vi "Scan.vi"() -> ()   [LabVIEW 2015]
uses:
  oskar_tools/seq_line.ctl
  oskar_tools/oskar_tools.lvlib
panel:
  in  "Open Button":bool
  in  "Make":bool
  in  "Tab Control":enum32{"Template", "Values", "Output", "README"}(tab)
  in  "Template":T1 caption="Template (placeholder: MOD)"
  in  "build mode":enum32{"step", "array"}(radio)
  in  "Shuffle":bool
  in  "Build Array":bool
  out "Array":string[](array[string])
  in  "Step":dbl=0.1
  in  "Stop":dbl=1.0
  in  "Start":dbl
  in  "Array size":i32=11
  in  "format string":string="%.4g"
  in  "SEQs":T1[](array[typedef])
  in  "Template":T1[](array[typedef])
  out "#":i32
  in  "Save":path
  in  "Stop Button":bool
  in  "Save Button":bool
  in  "Send Button":bool
  in  "New Button":bool
  # "Scan"
  # "### Overview ###\n\nCreate a sequence file that scans a VAR value over a linear series.\n\n### Instructions ###\n\nLoad or create a template sequence, using \"MOD\" in place of the value of the VAR to scan.\n\nOn the \"Values\" tab, build an array to cover the values that the VAR should take during the measurement.\n\nPress \"Make\" to create the sequence.  \"Save\" as a *.jsq file and \"Send\" it to sequencer.vi."
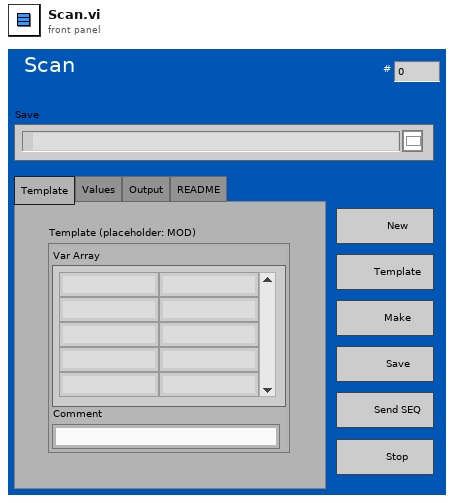
[diagram p1: front panel]
types:
  T1 = typedef "oskar_tools.lvlib/seq_line.ctl" = cluster{"Var Array":string[][], "Comment":string}
  T2 = enum8{"Enabled", "Disabled", "Disabled and Grayed Out"}
  T3 = enum16{"Left Button", "Center Button", "Right Button", "Window Close"}
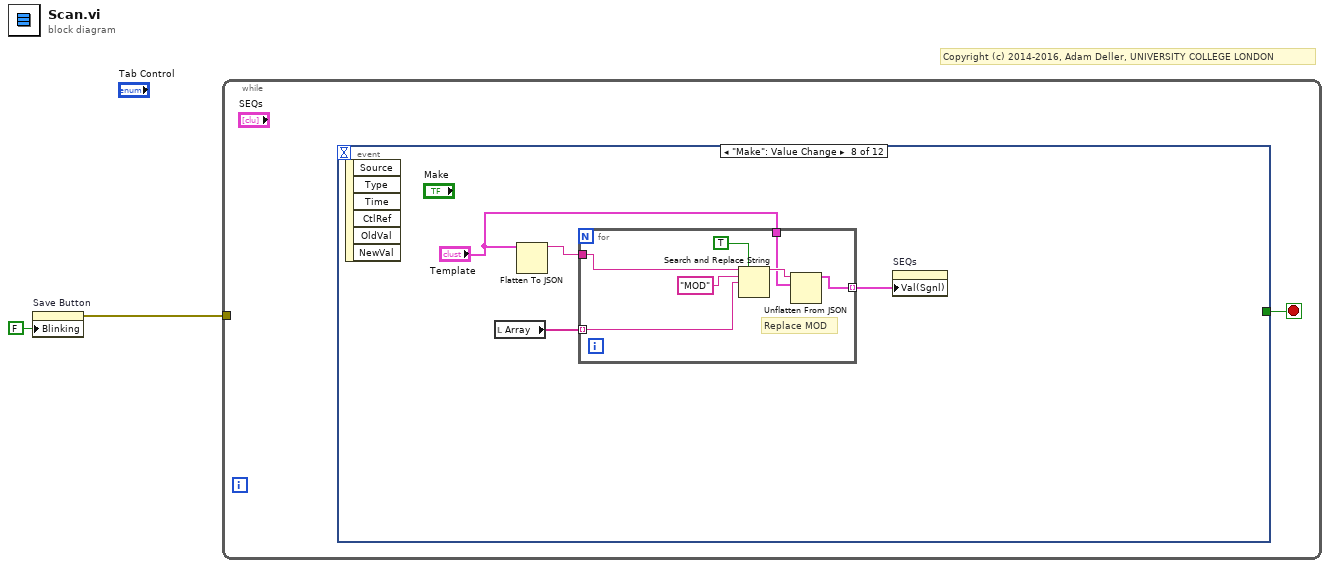
[diagram p0: block diagram]
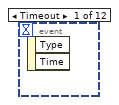
[diagram p2: hidden frame]
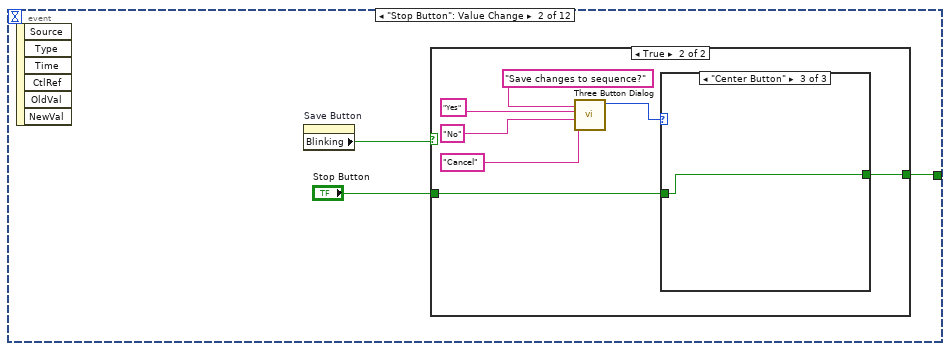
[diagram p3: hidden frame]
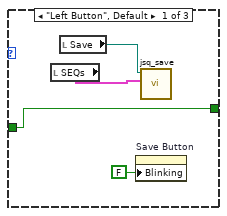
[diagram p5: hidden frame]
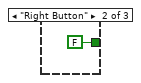
[diagram p6: hidden frame]
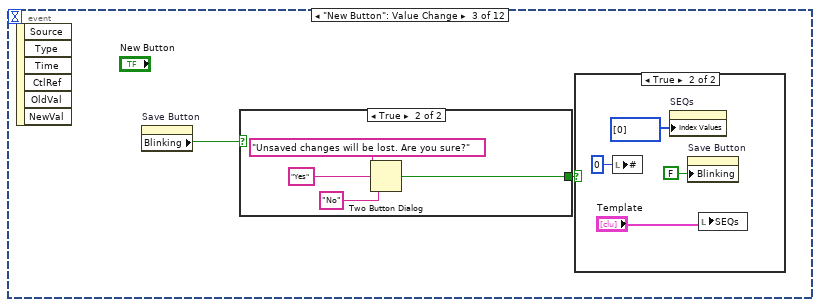
[diagram p7: hidden frame]
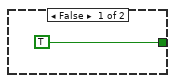
[diagram p9: hidden frame]
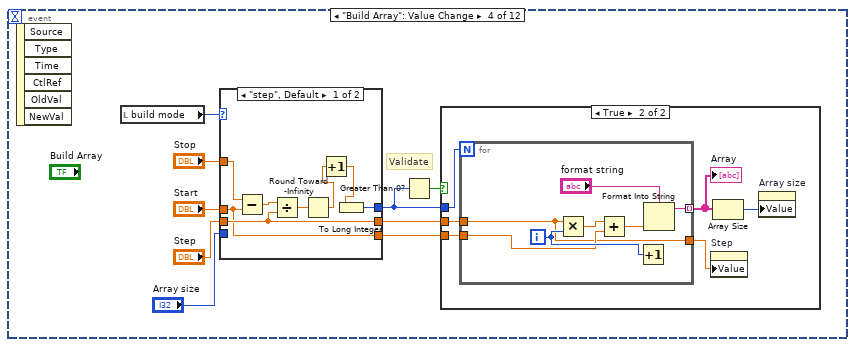
[diagram p10: hidden frame]
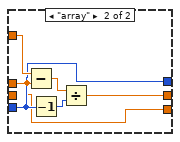
[diagram p11: hidden frame]
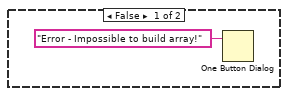
[diagram p12: hidden frame]
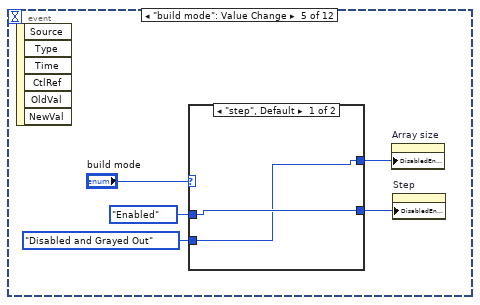
[diagram p13: hidden frame]
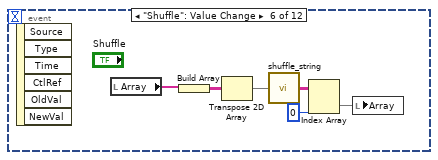
[diagram p15: hidden frame]
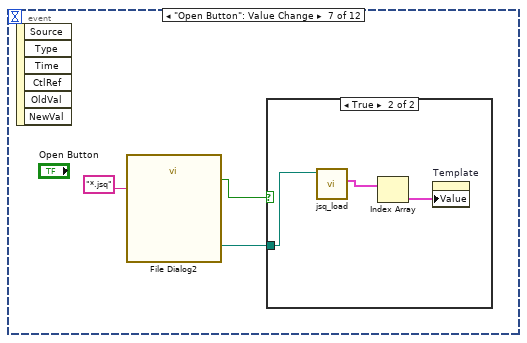
[diagram p16: hidden frame]
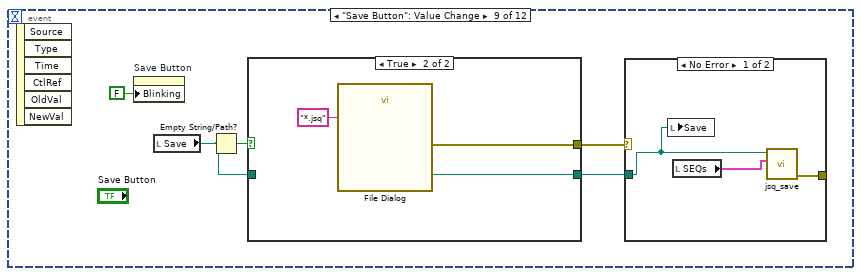
[diagram p18: hidden frame]
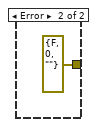
[diagram p19: hidden frame]
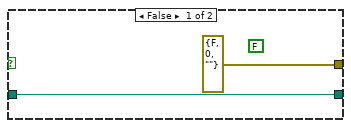
[diagram p20: hidden frame]
diagram:
  # "Copyright (c) 2014-2016, Adam Deller, UNIVERSITY COLLEGE LONDON"
  n1 = property on="Save Button" class="Bool"("Blinking"=FALSE) -> (error out=w1:errorcluster)  [unwired: 2 in, 1 out]
  n2 = while {
    tunnel: w1 -> [_]
    stop <- w3 stop-if-true
    n3 = event shown="[7] \"Make\": Value Change" {
      selector: _ -> [_ _ _ _ _ _ _ _ _ _ _ _]
      dyn-events: _ -> [_ _ _ _ _ _ _ _ _ _ _ _]
      timeout: _ -> [_ _ _ _ _ _ _ _ _ _ _ _]
      tunnel: [_ w6 _ _ _ _ _ _ _ _ _ _] -> w3
      event Timeout {
        n4 = event-data() -> ()  [unwired: 1 in, 2 out]
      }
      event "Stop Button": Value Change {
        n5 = event-data() -> ()  [unwired: 1 in, 6 out]
        n6 = property on="Save Button" class="Bool"() -> ("Blinking"=w5:bool)  [unwired: 2 in, 2 out]
        n7 = case shown="True" w5 {
          tunnel: [w7 w8] -> w6
          tunnel: "Stop Button" -> [w7 w9]
          frame False {
          }
          frame True {
            n8 = call <vilib>:"Three Button Dialog.vi"("Right Button Text (\"Cancel\")"="Cancel" ("Right Button Text (\"Cancel\")"), "Center Button Text (\"No\")"="No" ("F button name (\"Cancel\")"), "Left Button Text (\"Yes\")"="Yes" ("T button name (\"OK\")"), "message"="Save changes to sequence?") -> ("Which Button?"=w10:T3)  [unwired: 7 in]
            n9 = case shown="\"Center Button\"" w10 {
              tunnel: w9 -> [w18 _ w20]
              tunnel: [w18 FALSE ("Stop Button") w20] -> w8
              frame "Left Button", Default {
                n10 = local read "SEQs"() -> (w15:T1[])
                n11 = local read "Save"() -> (w17:path)
                n12 = property on="Save Button" class="Bool"("Blinking"=FALSE) -> ()  [unwired: 2 in, 2 out]
                n13 = call "jsq_save.vi"("SEQs"=w15, "Path"=w17) -> ()  [unwired: 7 in, 3 out]
              }
              frame "Right Button" {
              }
              frame "Center Button" {
              }
            }
          }
        }
      }
      event "New Button": Value Change {
        n14 = event-data() -> ()  [unwired: 1 in, 6 out]
        n15 = property on="Save Button" class="Bool"() -> ("Blinking"=w21:bool)  [unwired: 2 in, 2 out]
        n16 = case shown="True" w21 {
          tunnel: [TRUE w28] -> w22
          frame False {
          }
          frame True {
            n17 = Two Button Dialog(message="Unsaved changes will be lost. Are you sure?", 1:"No" ("F button name (\"Cancel\")"), 2:"Yes" ("T button name (\"OK\")")) -> (T button?=w28:bool)
          }
        }
        n18 = case shown="True" w22 {
          frame False {
          }
          frame True {
            n19 = local write "#"(0 ("#")) -> ()
            n20 = property on="SEQs" class="Arr (strict)"("Index Values"=u32[] [0]) -> ()  [unwired: 2 in, 2 out]
            n21 = property on="Save Button" class="Bool"("Blinking"=FALSE) -> ()  [unwired: 2 in, 2 out]
            n22 = local write "SEQs"("Template") -> ()
          }
        }
      }
      event "Build Array": Value Change {
        # "Validate"
        n23 = event-data() -> ()  [unwired: 1 in, 6 out]
        n24 = local read "build mode"() -> (w33:enum32{"step", "array"})
        n25 = case shown="\"step\", Default" w33 {
          tunnel: "Step" -> [w45 _]
          tunnel: "Stop" -> [w44 w53]
          tunnel: [w43 w49] -> w38
          tunnel: "Start" -> [w43 w49]
          tunnel: "Array size" -> [_ w50]
          tunnel: [w45 w52] -> w37
          tunnel: [w47 w50] -> w39
          frame "step", Default {
            n26 = Subtract(x=w44, y=w43) -> (x-y=w48:dbl)
            n27 = Divide(x=w48, y=w45) -> (x/y=w46:dbl)
            n28 = Round Toward -Infinity(1:w46) -> (0:w42:dbl)
            n29 = Increment(x=w42) -> (x+1=w41:dbl)
            n30 = To Long Integer(number=w41) -> (32bit integer=w47:i32)
          }
          frame "array" {
            n31 = Subtract(x=w53, y=w49) -> (x-y=w54:dbl)
            n32 = Decrement(x=w50) -> (x-1=w51:i32)
            n33 = Divide(x=w54, y=w51) -> (x/y=w52:dbl)
          }
        }
        n34 = Greater Than 0?(x=w39) -> (x > 0?=w40:bool)
        n35 = case shown="True" w40 {
          tunnel: w38 -> [_ w61]
          tunnel: w37 -> [_ w58]
          tunnel: w39 -> [_ w57]
          frame False {
            n36 = One Button Dialog(message="Error - Impossible to build array!") -> ()  [unwired: 1 in, 1 out]
          }
          frame True {
            n37 = for {
              N: w57 -> [_]
              tunnel: w61 -> [w64]
              tunnel: [w65] -> w60 mode=indexing
              tunnel: w58 -> [w62]
              tunnel: [w62] -> w56
              i -> [w68]
              n38 = Multiply(x=w62, y=w68) -> (x*y=w63:dbl)
              n39 = Add(x=w63, y=w64) -> (x+y=w66:dbl)
              n40 = Increment(x=w68) -> ()  [unwired: 1 out]
              n41 = Format Into String(format string="format string", w66) -> (resulting string=w65:string)  [unwired: 2 in, 1 out]
            }
            "Array" <- w60
            n42 = property on="Step" class="DigNum (strict)"("Value"=w56) -> ()  [unwired: 2 in, 2 out]
            n43 = Array Size(array=w60) -> (size(s)=w59:i32)
            n44 = property on="Array size" class="DigNum (strict)"("Value"=w59) -> ()  [unwired: 2 in, 2 out]
          }
        }
      }
      event "build mode": Value Change {
        n45 = event-data() -> ()  [unwired: 1 in, 6 out]
        n46 = case shown="\"step\", Default" "build mode" {
          tunnel: [w74 w77] -> w72
          tunnel: T2."Enabled" ("Disabled") -> [w75 w77]
          tunnel: [w75 w76] -> w70
          tunnel: T2."Disabled and Grayed Out" ("Disabled") -> [w74 w76]
          frame "step", Default {
          }
          frame "array" {
          }
        }
        n47 = property on="Array size" class="DigNum (strict)"("DisabledEnum"=w72) -> ()  [unwired: 2 in, 2 out]
        n48 = property on="Step" class="DigNum (strict)"("DisabledEnum"=w70) -> ()  [unwired: 2 in, 2 out]
      }
      event "Shuffle": Value Change {
        n49 = event-data() -> ()  [unwired: 1 in, 6 out]
        n50 = local read "Array"() -> (w83:string[])
        n51 = Build Array(w83) -> (w80:string[][])
        n52 = Transpose 2D Array(2D array=w80) -> (transposed array=w79:string[][])
        n53 = call "shuffle_string.vi"("Array IN"=w79) -> ("Array OUT"=w82:string[][])
        n54 = Index Array(array=w82, index (col)=0 ("disabled index (col)")) -> (element=w81:string[])  [unwired: 1 in]
        n55 = local write "Array"(w81) -> ()
      }
      event "Open Button": Value Change {
        n56 = event-data() -> ()  [unwired: 1 in, 6 out]
        n57 = call "File Dialog2"("pattern (all files)"="*.jsq") -> ("selected path"=w85:path, "exists"=w86:bool)  [unwired: 11 in, 2 out]
        n58 = case shown="True" w86 {
          tunnel: w85 -> [_ w89]
          frame False {
          }
          frame True {
            n59 = call "jsq_load.vi"("Open"=w89) -> ("SEQs"=w88:T1[])  [unwired: 7 in, 3 out]
            n60 = Index Array(array=w88) -> (element=w87:T1)  [unwired: 1 in]
            n61 = property on="Template" class="Clust (strict)"("Value"=w87) -> ()  [unwired: 2 in, 2 out]
          }
        }
      }
      event "Make": Value Change {
        n62 = event-data() -> ()  [unwired: 1 in, 6 out]
        n63 = local read "Array"() -> (w92:string[])
        n64 = Flatten To JSON(anything="Template") -> (JSON string=w93:string)  [unwired: 2 in, 1 out]
        n65 = for {
          tunnel: w93 -> [w99]
          tunnel: w92 -> [w97] mode=indexing
          tunnel: [w94] -> w90 mode=indexing
          tunnel: "Template" -> [w95]
          # "Replace MOD"
          n66 = Search and Replace String(replace all?=TRUE ("replace all? (F)"), input string=w99, search string="MOD", replace string=w97) -> (result string=w96:string)  [unwired: 4 in, 3 out]
          n67 = Unflatten From JSON(JSON string=w96, type and defaults=w95) -> (value=w94:T1)  [unwired: 5 in, 1 out]
        }
        n68 = property on="SEQs" class="Arr (strict)"("Val(Sgnl)"=w90) -> ()  [unwired: 2 in, 2 out]
      }
      event "Save Button": Value Change {
        n69 = event-data() -> ()  [unwired: 1 in, 6 out]
        n70 = property on="Save Button" class="Bool"("Blinking"=FALSE) -> ()  [unwired: 2 in, 2 out]
        n71 = local read "Save"() -> (w103:path)
        n72 = Empty String/Path?(string/path=w103) -> (empty?=w104:bool)
        n73 = case shown="True" w104 {
          tunnel: [w111 w114] -> w102
          tunnel: w103 -> [w111 _]
          tunnel: [errorcluster {"status"=FALSE, "code"=0, "source"=""} ("error out") w112] -> w101
          frame False {
            (unwired) FALSE ("cancelled")
          }
          frame True {
            n74 = call "File Dialog"("pattern (all files)"="*.jsq") -> ("selected path"=w114:path, "error out"=w112:errorcluster)  [unwired: 11 in, 2 out]
          }
        }
        n75 = case shown="No Error" w101 {
          tunnel: w102 -> [w107 _]
          tunnel: [w106 errorcluster {"status"=FALSE, "code"=0, "source"=""} ("error out")] -> _
          frame No Error {
            n76 = local write "Save"(w107) -> ()
            n77 = local read "SEQs"() -> (w108:T1[])
            n78 = call "jsq_save.vi"("SEQs"=w108, "Path"=w107) -> ("error out"=w106:errorcluster)  [unwired: 7 in, 2 out]
          }
          frame Error {
          }
        }
      }
      event "Save": Value Change {
        n79 = event-data() -> ()  [unwired: 1 in, 6 out]
        n80 = property on="Save Button" class="Bool"("Blinking"=TRUE) -> ()  [unwired: 2 in, 2 out]
      }
      event "SEQs": Value Change {
        n81 = event-data() -> ("NewVal"=w117:T1[])  [unwired: 1 in, 5 out]
        n82 = Array Size(array=w117) -> (size(s)=→"#":i32)
        n83 = property on="Save Button" class="Bool"("Blinking"=TRUE) -> ()  [unwired: 2 in, 2 out]
      }
      event "Send Button": Value Change {
        n84 = event-data() -> ()  [unwired: 1 in, 5 out]
        n85 = property on="Save Button" class="Bool"() -> ("Blinking"=w120:bool)  [unwired: 2 in, 2 out]
        n86 = case shown="False" w120 {
          tunnel: [TRUE w123] -> w119
          frame False {
          }
          frame True {
            n87 = Two Button Dialog(message="This sequence has not been saved.  Load saved version into sequencer?", 1:"Cancel" ("F button name (\"Cancel\")"), 2:"Ok" ("T button name (\"OK\")")) -> (T button?=w123:bool)
          }
        }
        n88 = case shown="True" w119 {
          frame False {
          }
          frame True {
            n89 = call "jsq_send.vi"("Sequence File"="Save") -> ()  [unwired: 11 in]
          }
        }
      }
    }
  }
